vi "Advanced Serial Write and Read.vi"(0 "VISA resource name":refnum<visa-resource-name>="COM1" caption="VISA资源名称", 1 "baud rate":u32=9600 caption="波特率", 3 "bytes to read":u32=1000 caption="读取的字节", 4 "data bits":u16=8 caption="数据比特" min=5 max=8 step=1, 5 "parity":u16(ring) caption="奇偶" items=["无", "奇", "偶", "标记", "空格"], 7 "stop bits":u16(ring)=10 caption="停止位" items=["1.0"=10, "1.5"=15, "2.0"=20], 9 "XON Character":u8=17 caption="XON字符" format="%.0x", 13 "string to write":string="*IDN?" caption="写入字符串", 14 "XOFF Character":u8=19 caption="XOFF字符" format="%.0x", 15 "timeout (ms)":u32=10000 caption="超时(ms)", 17 "write":bool=TRUE caption="写入", 21 "End read on termination character?":bool=TRUE caption="终止符时结束读取？", 24 "termination char\n(0xA = '\\n' = LF)":u8=10 caption="终止符\n(0xA = '\\n' = LF)" format="%.0x", 25 "Input\nbuffer size":u32=4096 caption="输入\n缓冲区大小", 26 "read":bool=TRUE caption="读取") -> (20 "read string":string caption="读取字符串")   [LabVIEW 2010]
doc: "高级串行读取和写入范例可执行串口读取、串口写入或者串口读写操作，同时可设置串口高级功能，例如缓冲区大小、终止符和XON/XOFF流控制等。用户可在前面板选择操作（读取或写入）。如果选择全部，VI将写入数据并读取数据，然后关闭开放给端口的VISA会话句柄。\n\n串口的参数组必须匹配连接仪器或设备的参数。在本范例中，待读取字节参数可指定串口读取的字节数。如端口字节超过指定的字节数，超出部分将不会被读取。如果指定读取的字节数超过实际字节数，可能返回超时错误。\n\n步骤：\n1) 选择串行资源并配置参数（波特率、数据位、奇偶、停止位和流控制）。\n2) 可以启用并设置终止符。运行本范例前先设置所需输入缓冲区大小。\n3) 选择需执行的操作。\n4) 连接串口至设备。如未发现可用设备，请按以下任一方式执行环回测试。在RS-232线缆中短路引脚2和3，或者在RS-485/422线缆中短路引脚4和8以及引脚5和9。\n5) 运行VI并查看读取的数据。（如果已执行环回测试，“读取字符串”将匹配“写入字符串”。）\n\n本范例说明的部分高级功能可能有利于用户的应用程序开发。应用程序并不需要使用范例中的全部功能。设置输入缓冲区大小对应用程序十分重要。本范例可扩展流控制选项以包括XON和XOFF，从而允许用户选择控制字符。在前面板中显示超时参数，以便于用户指定VISA读取等待指定字节数的超时时间。同时用户可使用多种方式控制结束符，请查看后续说明。\n\n请注意在运行范例时，用户可以单击写入或读取按钮并更改读取字节参数的值。但对于其它参数，必须先停止该范例才能进行修改。\n\n将I/O缓冲区大小设置为超出预期接收数据总数。这将有利于不使用流控制的应用程序，因为当接收缓冲区溢出时可能会丢失字符。\n\n设置超时时间，确保当操作在指定时间内无法完成时可返回一个超时错误。\n\n部分设备需要通过终止符确定命令字符串的结束位置。部分设备将发送终止符以说明待读取数据的末端。\n\n本范例将说明当缓冲区中发现结束符时如何结束读取操作或者添加结束符至写入数据的末端。如需启用读取至终止符，可使用“VISA配置串口”函数或者用于读取、结束符启用和结束符的VISA属性串口结束模式。如需使用终止符结束写入，可使用写入、发送结束启用和结束符的VISA属性串口结束模式。在本范例中，读取和写入操作将使用相同的终止符。在应用程序中也可以指定两个不同的终止符。\n\n用户的应用程序可能需要特定字符用于XON/XOFF流控制。通过VISA属性流控制XOFF字符和流控制XON字符可以指定该字符。请注意如使用标准XON和XOFF字符，无法将十进制17和19作为数据值。同时使用流控制并设置正确的缓冲区大小可避免缓冲区溢出。"
uses:
  <vilib>/Instr/_visa.llb/VISA Configure Serial Port (Instr).vi
panel:
  out "actual bytes read":u32 caption="实际字节读取"
  in  "stop":bool caption="停止"
  in  "flow control":u16(ring) caption="流程控制" items=["无"=0, "XON/XOFF"=1, "RTS/CTS"=2, "DTR/DSR"=4]
  in  "End write with termination character?":bool=TRUE caption="终止符时结束写入？"
  # "Windows/Linux用户可使用仪器驱动查找器（帮助>>查找仪器驱动程序）为仪器查找相应的驱动程序。"
  # "选择串口资源以及执行的操作。如果选择全部，VI将写入数据并读取数据，然后关闭开放给端口的VISA会话句柄。该VI将等待直到端口接收到指定的字节数、出现超时，或者接收到终止符。本范例中的默认终止符为换行符( ASCII 0xA, '\\n' )。运行本范例前先设置所需输入缓冲区大小。\n注：该范例将在单击“停止”按钮前连续执行循环。"
  # "更多信息请选择文件>>VI属性>>说明信息"
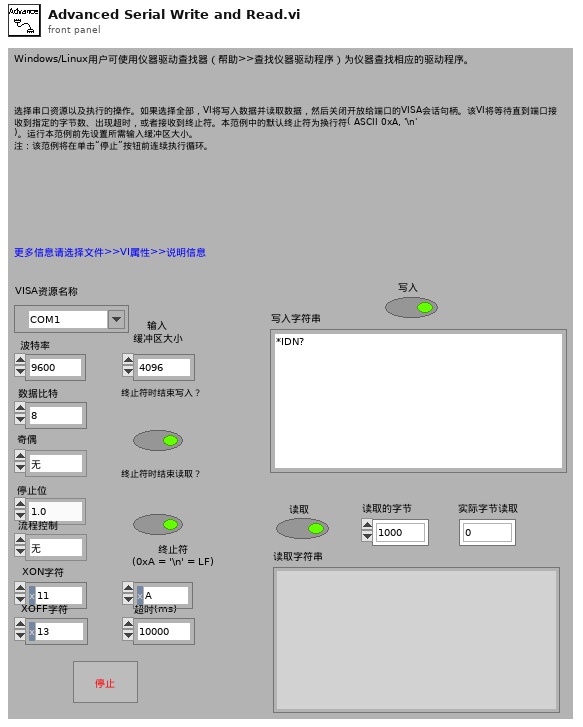
[diagram p1: front panel]
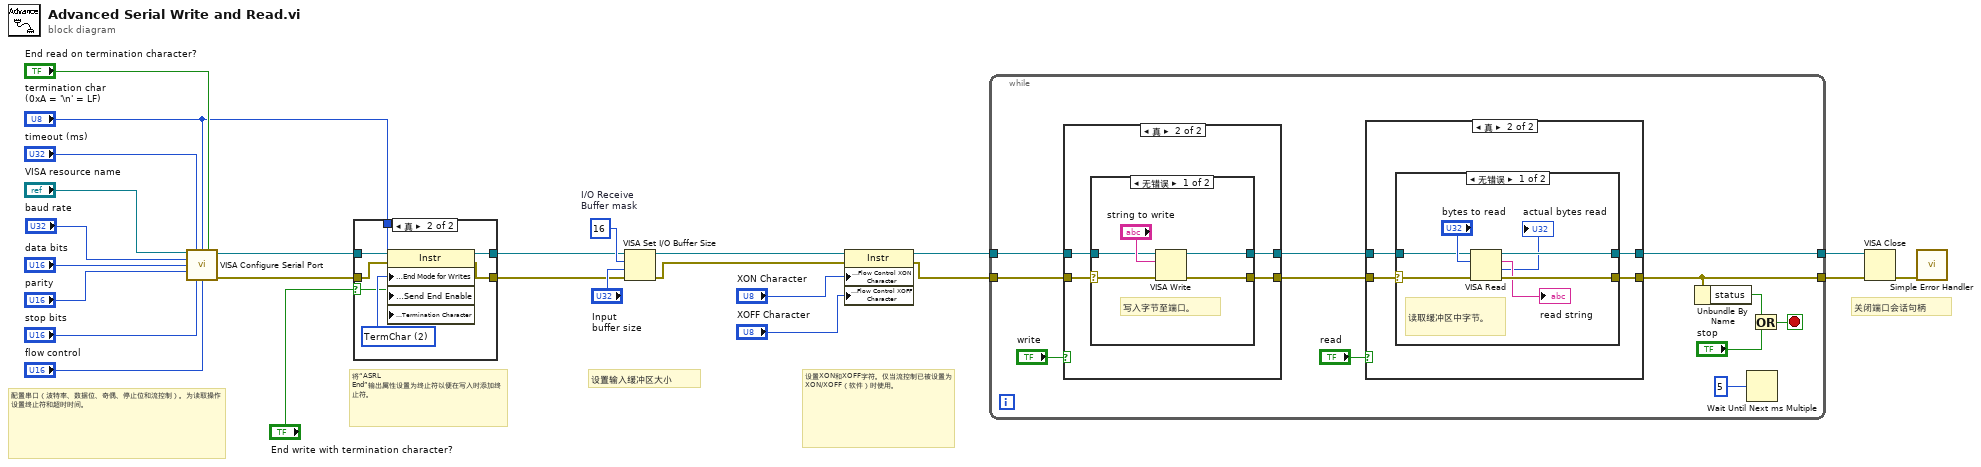
[diagram p0: block diagram]
diagram:
  w18 = u16 16  # I/O Receive Buffer mask
  # "设置XON和XOFF字符。仅当流控制已被设置为XON/XOFF（软件）时使用。"
  # "配置串口（波特率、数据位、奇偶、停止位和流控制）。为读取操作设置终止符和超时时间。"
  # "设置输入缓冲区大小"
  # "将“ASRL End”输出属性设置为终止符以便在写入时添加终止符。"
  # "关闭端口会话句柄"
  n1 = call-poly "VISA Configure Serial Port"("VISA resource name"="VISA resource name", "timeout (10sec)"="timeout (ms)", "termination char\n(0xA = '\\n' = LF)"="termination char\n(0xA = '\\n' = LF)", "Enable Termination\nChar (T)"="End read on termination character?", "baud rate (9600)"="baud rate", "data bits (8)"="data bits", "parity (0:none)"="parity", "stop bits (10: 1 bit)"="stop bits", "flow control (0:none)"="flow control") -> ("VISA resource name out"=w4:refnum<visa-resource-name>, "error out"=w7:errorcluster)  [unwired: 1 in, 4 out]
  n2 = case shown="真" "End write with termination character?" {
    selector: "End write with termination character?" -> [_ w28]
    tunnel: w4 -> [w26 w34]
    tunnel: w7 -> [w27 w33]
    tunnel: [w26 w32] -> w5
    tunnel: [w27 w31] -> w6
    tunnel: "termination char\n(0xA = '\\n' = LF)" -> [_ w29]
    frame False {
    }
    frame True {
      w30 = u16 2 items=["None", "LastBit", "TermChar", "Break"] ("Serial Settings:Serial End Mode for Writes")
      n3 = property class="Instr"(reference=w34, error in=w33, "Serial Settings:End Mode for Writes"=w30, "Message Based Settings:Send End Enable"=w28, "Message Based Settings:Termination Character"=w29) -> (reference out=w32:refnum<visa-resource-name>, error out=w31:errorcluster)
    }
  }
  n4 = VISA Set I/O Buffer Size(VISA resource name=w5, mask (16)=w18, size (4096)="Input\nbuffer size", error in (no error)=w6) -> (VISA resource name out=w13:refnum<visa-resource-name>, error out=w12:errorcluster)
  n5 = property class="Instr"(reference=w13, error in=w12, "Serial Settings:Flow Control XON Character"="XON Character", "Serial Settings:Flow Control XOFF Character"="XOFF Character") -> (reference out=w3:refnum<visa-resource-name>, error out=w9:errorcluster)
  n6 = while {
    tunnel: w9 -> [w39]
    tunnel: w3 -> [w40]
    tunnel: [w38] -> w2
    tunnel: [w37] -> w1
    stop <- w36 stop-if-true
    n7 = case shown="真" "write" {
      tunnel: [w48 w52] -> w43
      tunnel: [w47 w51] -> w42
      tunnel: w40 -> [w48 w50]
      tunnel: w39 -> [w47 w49]
      frame False {
      }
      frame True {
        n8 = case shown="无错误" w49 {
          selector: w49 -> [w53 w59]
          tunnel: [w57 w58] -> w52
          tunnel: [w56 w59] -> w51
          tunnel: w50 -> [w54 w58]
          frame No Error {
            # "写入字节至端口。"
            n9 = VISA Write(VISA resource name=w54, write buffer="string to write", error in (no error)=w53) -> (VISA resource name out=w57:refnum<visa-resource-name>, error out=w56:errorcluster)  [unwired: 1 out]
          }
          frame Error {
          }
        }
      }
    }
    n10 = case shown="真" "read" {
      tunnel: w42 -> [w60 w63]
      tunnel: w43 -> [w61 w62]
      tunnel: [w60 w65] -> w37
      tunnel: [w61 w64] -> w38
      frame False {
      }
      frame True {
        n11 = case "Read bytes from port." shown="无错误" w63 {
          selector: w63 -> [w67 w73]
          tunnel: [w71 w73] -> w65
          tunnel: [w72 w74] -> w64
          tunnel: w62 -> [w68 w74]
          frame No Error {
            # "读取缓冲区中字节。"
            n12 = VISA Read(VISA resource name=w68, byte count="bytes to read", error in (no error)=w67) -> (VISA resource name out=w72:refnum<visa-resource-name>, read buffer=→"read string":string, return count=→"actual bytes read":u32, error out=w71:errorcluster)
          }
          frame Error {
            # "在串口读取\n字节时发生\n错误"
          }
        }
      }
    }
    n13 = Unbundle By Name(w37) -> ("status"=w44:bool)
    n14 = Wait Until Next ms Multiple(millisecond multiple=u32 5) -> ()  [unwired: 1 out]
    n15 = Or(x=w44, y="stop") -> (x .or. y?=w36:bool)
  }
  n16 = VISA Close(VISA resource name=w2, error in (no error)=w1) -> (error out=w23:errorcluster)
  n17 = call <vilib>:"Simple Error Handler.vi"("error in (no error)"=w23) -> ()  [unwired: 1 in, 8 out]
